vi "CallByRefParallel Abort.vi"(8 "error in (no error)":errorcluster, 11 "VI Refnum":refnum<vi>) -> (0 "error out":errorcluster, 3 "VI Refnum dup":refnum<vi>)   [LabVIEW 2011, in "COSYLib.lvlib"]
doc: "Simple VI for aborting a VI."
uses:
  COSYLib.lvlib
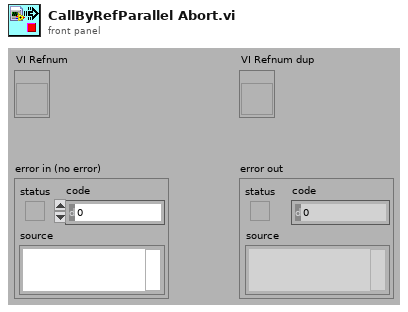
[diagram p1: front panel]
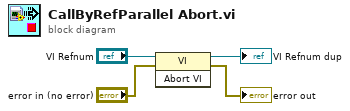
[diagram p0: block diagram]
diagram:
  n1 = invoke class="VI" method="Abort VI"(reference="VI Refnum", error in="error in (no error)") -> (reference out=→"VI Refnum dup":refnum<vi>, error out=→"error out":errorcluster)  [unwired: 1 in, 1 out]
